vi "Latch.vi"(11 "Latch In":bool) -> (3 "Latch Out":bool)   [LabVIEW 2012]
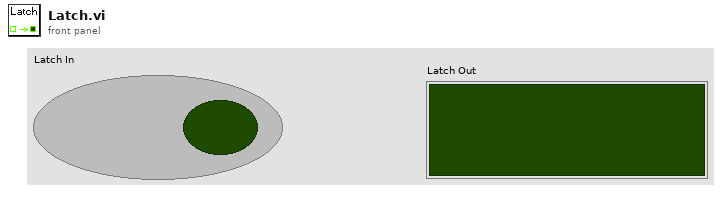
[diagram p1: front panel]
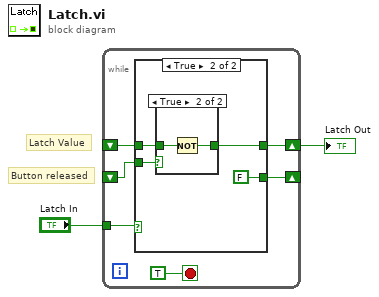
[diagram p0: block diagram]
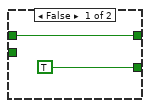
[diagram p2: hidden frame]
diagram:
  # "Latch Value"
  # "Button released"
  n1 = while {
    tunnel: "Latch In" -> [w7]
    shift-right: [w6] -> _
    shift-left: _ -> [w3]
    shift-right: [w5] -> w1
    shift-left: _ -> [w4]
    stop <- TRUE stop-if-true
    n2 = case shown="True" w7 {
      tunnel: [TRUE FALSE] -> w6
      tunnel: [w9 w13] -> w5
      tunnel: w4 -> [w9 w12]
      tunnel: w3 -> [_ w11]
      frame False {
      }
      frame True {
        n3 = case shown="True" w11 {
          tunnel: [w15 w17] -> w13
          tunnel: w12 -> [w15 w16]
          frame False {
          }
          frame True {
            n4 = Not(x=w16) -> (.not. x?=w17:bool)
          }
        }
      }
    }
  }
  "Latch Out" <- w1
